vi "PathOptimization.vi"(9 "Joint 2 Angle":dbl[](array[numeric])=[286.0, 151.0], 10 "Joint 1 Angle":dbl[](array[numeric])=[164.0, 117.0]) -> (1 "subarray joint 2":dbl[](array[numeric]), 2 "subarray joint 1":dbl[](array[numeric]))   [LabVIEW 2023]
uses:
  Framework/Robot Global Data.vi
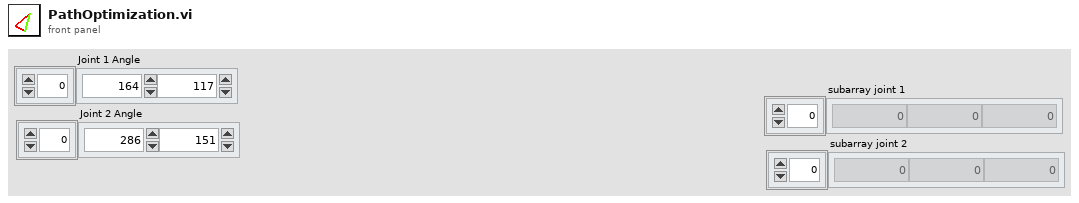
[diagram p1: front panel]
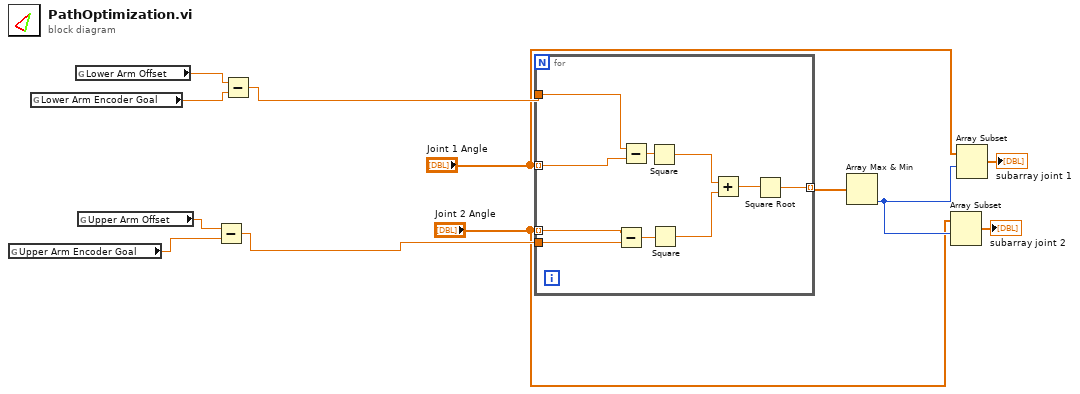
[diagram p0: block diagram]
diagram:
  n1 = global read "Robot Global Data.vi" "Upper Arm Encoder Goal"() -> (w2:dbl)
  n2 = global read "Robot Global Data.vi" "Lower Arm Encoder Goal"() -> (w3:dbl)
  n3 = global read "Robot Global Data.vi" "Lower Arm Offset"() -> (w4:dbl)
  n4 = global read "Robot Global Data.vi" "Upper Arm Offset"() -> (w1:dbl)
  n5 = Subtract(x=w1, y=w2) -> (x-y=w11:dbl)
  n6 = Subtract(x=w4, y=w3) -> (x-y=w12:dbl)
  n7 = for {
    tunnel: "Joint 1 Angle" -> [w22] mode=indexing
    tunnel: "Joint 2 Angle" -> [w19] mode=indexing
    tunnel: w12 -> [w21]
    tunnel: w11 -> [w18]
    tunnel: [w13] -> w10 mode=indexing
    n8 = Subtract(x=w19, y=w18) -> (x-y=w17:dbl)
    n9 = Subtract(x=w21, y=w22) -> (x-y=w20:dbl)
    n10 = Square(x=w20) -> (x^2=w16:dbl)
    n11 = Square(x=w17) -> (x^2=w15:dbl)
    n12 = Add(x=w16, y=w15) -> (x+y=w14:dbl)
    n13 = Square Root(x=w14) -> (sqrt(x)=w13:dbl)
  }
  n14 = Array Max & Min(array=w10) -> (min index (indices)=w9:i32)  [unwired: 3 out]
  n15 = Array Subset(array="Joint 2 Angle", index=w9) -> (→"subarray joint 2":dbl[])  [unwired: 1 in]
  n16 = Array Subset(array="Joint 1 Angle", index=w9) -> (→"subarray joint 1":dbl[])  [unwired: 1 in]
